vi "Supervisor Chat.vi"(9 "Stop Chat":bool, 10 "Send":bool, 11 "Enter Text":string) -> (3 "Chat Window":string)   [LabVIEW 2017]
uses:
  <vilib>/OPCUA/controls/Write Status.ctl
  <vilib>/OPCUA/controls/NodeId.ctl
  <vilib>/OPCUA/client/Multiple Write String.vi
  <vilib>/OPCUA/NI OPC UA Client.lvlib
panel:
  out "Log Loop":i32
  out "Send Loop":i32
  in  "Node Status":T1 items=["Good"=0, "Uncertain_InitialValue"=1083310080, "Uncertain_LastUsableValue"=1083179008, "Uncertain_SensorNotAccurate"=1083375616, "Uncertain_EngineeringUnitsExceeded"=1083441152, "Bad_NoCommunication"=2150694912, "Bad_NotReadable"=2151284736, "Bad_NotWritable"=2151350272, "Bad_OutOfRange"=2151415808, "Bad_WaitingForInitialData"=2150760448]
  in  "Time Stamp":timestamp
  in  "Node Status":T1 items=["Good"=0, "Uncertain_InitialValue"=1083310080, "Uncertain_LastUsableValue"=1083179008, "Uncertain_SensorNotAccurate"=1083375616, "Uncertain_EngineeringUnitsExceeded"=1083441152, "Bad_NoCommunication"=2150694912, "Bad_NotReadable"=2151284736, "Bad_NotWritable"=2151350272, "Bad_OutOfRange"=2151415808, "Bad_WaitingForInitialData"=2150760448]
  in  "Time Stamp":timestamp
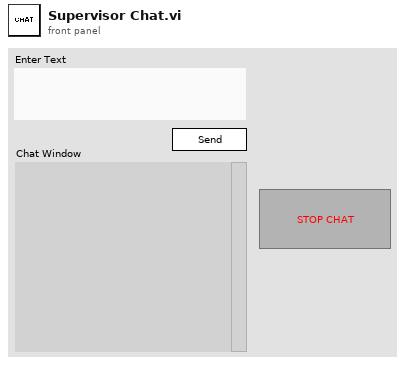
[diagram p1: front panel]
types:
  T1 = typedef "Write Status.ctl" = u32
  T2 = enum16{"open", "replace", "create", "open or create", "replace or create", "replace or create with confirmation"}
  T3 = typedef "OPC UA Client Refnum.ctl" = refnum<k21>
  T4 = typedef "NodeId.ctl" = string
  T5 = cluster{"node ID":T4, "value":string, "timestamp (current time)":timestamp, "node status":T1}
  T6 = cluster{"node ID":T4, "value":string, "timestamp (current time)":timestamp, "node status":T1}[]
  T7 = typedef "Subscription ID.ctl" = u32
  T8 = typedef "Subscription Data Change.ctl" = cluster{"node ID":T4, " value":variant, "timestamp":timestamp, "data type":T9, "status code":T10}
  T9 = typedef "Data Type.ctl" = u16
  T10 = typedef "OPC UA StatusCode.ctl" = u32
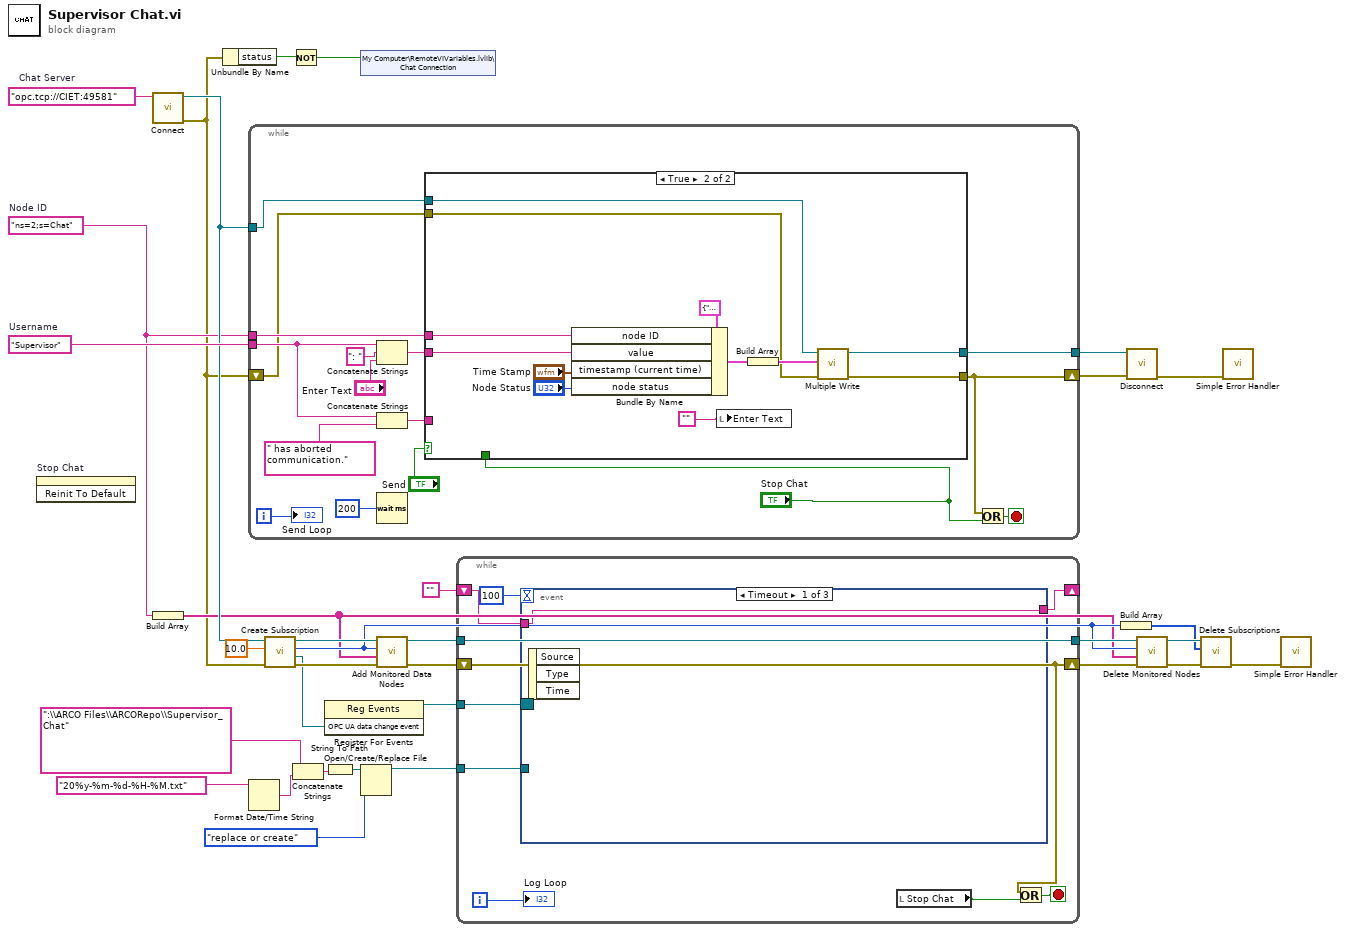
[diagram p0: block diagram]
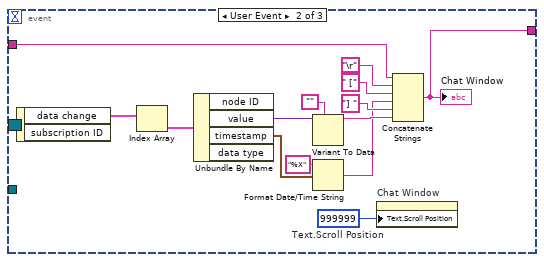
[diagram p2: hidden frame]
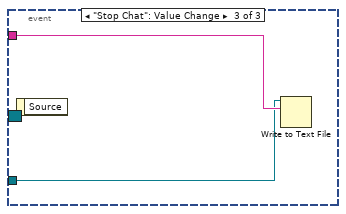
[diagram p3: hidden frame]
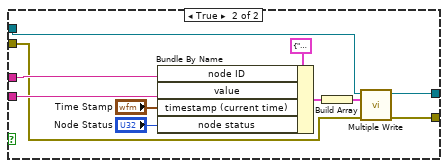
[diagram p5: hidden frame]
diagram:
  w15 = "ns=2;s=Chat"  # Node ID
  w31 = "Supervisor"  # Username
  w32 = "opc.tcp://CIET:49581"  # Chat Server
  n1 = invoke on="Stop Chat" class="Bool (strict)" method="Reinit To Default"() -> ()  [unwired: 3 in, 3 out]
  n2 = call <vilib>:"Connect.vi"("server endpoint URL"=w32) -> ("error out"=w3:errorcluster, "OPC UA client refnum out"=w30:T3)  [unwired: 8 in, 1 out]
  n3 = Build Array(w15) -> (w14:string[])
  n4 = Unbundle By Name(w3) -> ("status"=w5:bool)
  n5 = while {
    tunnel: w15 -> [w41]
    tunnel: w31 -> [w46]
    tunnel: w30 -> [w39]
    tunnel: [w40] -> w12
    shift-right: [w34] -> w2
    shift-left: w3 -> [w38]
    i -> [w44]
    stop <- w36 stop-if-true
    n6 = Concatenate Strings(w46, ": ", "Enter Text") -> (w42:string)
    n7 = Concatenate Strings(w46, " has aborted communication.") -> (w37:string)
    n8 = Wait (ms)(milliseconds to wait=u32 200) -> ()  [unwired: 1 out]
    n9 = case shown="True" "Send" {
      tunnel: w42 -> [_ w76]
      tunnel: w41 -> [w54 w75]
      tunnel: [w50 w73] -> w40
      tunnel: [w51 w72] -> w34
      tunnel: w39 -> [w52 w71]
      tunnel: w38 -> [w53 w70]
      tunnel: "Stop Chat" -> [w56 _]
      tunnel: w37 -> [w55 _]
      frame False {
        n10 = case shown="False" w56 {
          tunnel: w55 -> [_ w64]
          tunnel: w54 -> [_ w63]
          tunnel: w53 -> [w57 w62]
          tunnel: w52 -> [w58 w61]
          tunnel: [w58 w60] -> w50
          tunnel: [w57 w59] -> w51
          frame False {
          }
          frame True {
            n11 = Bundle By Name(cluster=T5 {"node ID"="", "value"="", "timestamp (current time)"=timestamp(0 s since 1904-01-01), "node status"=0} ("request"), "node ID"=w63, "value"=w64, "timestamp (current time)"="Time Stamp", "node status"="Node Status") -> (w67:T5)
            n12 = Build Array(w67) -> (w66:T6)
            n13 = call-poly <vilib>:"Multiple Write.vi"("error in (no error)"=w62, "requests"=w66, "OPC UA client refnum in"=w61) -> ("error out"=w59:errorcluster, "OPC UA client refnum out"=w60:T3)  [unwired: 5 in, 2 out]
          }
        }
      }
      frame True {
        n14 = Bundle By Name(cluster=T5 {"node ID"="", "value"="", "timestamp (current time)"=timestamp(0 s since 1904-01-01), "node status"=0} ("request"), "node ID"=w75, "value"=w76, "timestamp (current time)"="Time Stamp", "node status"="Node Status") -> (w79:T5)
        n15 = local write "Enter Text"("") -> ()
        n16 = Build Array(w79) -> (w78:T6)
        n17 = call-poly <vilib>:"Multiple Write.vi"("error in (no error)"=w70, "requests"=w78, "OPC UA client refnum in"=w71) -> ("error out"=w72:errorcluster, "OPC UA client refnum out"=w73:T3)  [unwired: 5 in, 2 out]
      }
    }
    n18 = Or(x=w34, y="Stop Chat") -> (x .or. y?=w36:bool)
    "Send Loop" <- w44
  }
  n19 = Format Date/Time String(time format string (%c)="20%y-%m-%d-%H-%M.txt") -> (date/time string=w9:string)  [unwired: 2 in]
  n20 = call <vilib>:"Create Subscription.vi"("error in (no error)"=w3, "publishing interval (1000 ms)"=10.0, "OPC UA client refnum in"=w30) -> ("error out"=w28:errorcluster, "OPC UA data change event"=w27:refnum<user-event>, "subscription ID out"=w19:T7, "OPC UA client refnum out"=w29:T3)  [unwired: 4 in, 1 out]
  n21 = Not(x=w5) -> (.not. x?=w4:bool)
  n22 = Concatenate Strings(":\\ARCO Files\\ARCORepo\\Supervisor_Chat", w9) -> (w7:string)
  n23 = register-events(w27) -> (reference out=w26:refnum<event-registration>)  [unwired: 2 in, 1 out]
  n24 = String To Path(string=w7) -> (path=w6:path)
  n25 = shared-variable "My Computer\\RemoteVIVariables.lvlib\\Chat Connection"(w4) -> ()  [unwired: 1 in, 1 out]
  n26 = Open/Create/Replace File(file path (use dialog)=w6, operation (0:open)=T2."replace or create") -> (refnum out=w16:refnum<file>)  [unwired: 4 in, 2 out]
  n27 = call <vilib>:"Add Monitored Data Nodes.vi"("error in (no error)"=w28, "node IDs"=w14, "subscription ID in"=w19, "OPC UA client refnum in"=w29) -> ("error out"=w22:errorcluster, "OPC UA client refnum out"=w24:T3)  [unwired: 4 in, 2 out]
  n28 = while {
    tunnel: w26 -> [w91]
    shift-right: [w89] -> _
    shift-left: "" -> [w90]
    tunnel: w24 -> [w88]
    tunnel: [w88] -> w23
    tunnel: w16 -> [w87]
    shift-right: [w83] -> w1
    shift-left: w22 -> [w83]
    i -> [w86]
    stop <- w84 stop-if-true
    n29 = event shown="[0] Timeout" {
      selector: w91 -> [_ _ _]
      dyn-events: _ -> [_ _ _]
      timeout: 100 -> [_ _ _]
      tunnel: w90 -> [w92 w95 w108]
      tunnel: [w92 w94 _] -> w89
      tunnel: w87 -> [_ _ w107]
      event Timeout {
        n30 = event-data() -> ()  [unwired: 1 in, 3 out]
      }
      event User Event {
        w93 = u32 999999  # Text.Scroll Position
        n31 = event-data() -> ("data change"=w106:T8[])  [unwired: 1 in, 1 out]
        n32 = Index Array(array=w106) -> (element=w105:T8)  [unwired: 1 in]
        n33 = Unbundle By Name(w105) -> ("value"=w104:variant, "timestamp"=w102:timestamp)  [unwired: 2 out]
        n34 = Variant To Data(type="", Variant=w104) -> (data=w100:string)  [unwired: 1 in, 1 out]
        n35 = Format Date/Time String(time format string (%c)="%X", seconds (now)=w102) -> (date/time string=w98:string)  [unwired: 1 in]
        n36 = property on="Chat Window" class="Str"("Text.Scroll Position"=w93) -> ()  [unwired: 2 in, 2 out]
        n37 = Concatenate Strings(w95, "\r", " [", w98, "] ", w100) -> (w94:string)
        "Chat Window" <- w94
      }
      event "Stop Chat": Value Change {
        n38 = event-data() -> ()  [unwired: 1 in, 1 out]
        n39 = Write to Text File(file (use dialog)=w107, text=w108) -> ()  [unwired: 2 in, 3 out]
      }
    }
    n40 = local read "Stop Chat"() -> (w82:bool)
    n41 = Or(x=w83, y=w82) -> (x .or. y?=w84:bool)
    "Log Loop" <- w86
  }
  n42 = Build Array(w19) -> (w18:T7[])
  n43 = call <vilib>:"Disconnect.vi"("error in (no error)"=w2, "OPC UA client refnum in"=w12) -> ("error out"=w33:errorcluster)  [unwired: 9 in]
  n44 = call <vilib>:"Delete Monitored Nodes.vi"("error in (no error)"=w1, "node IDs"=w14, "subscription ID in"=w19, "OPC UA client refnum in"=w23) -> ("error out"=w20:errorcluster, "OPC UA client refnum out"=w21:T3)  [unwired: 3 in, 3 out]
  n45 = call <vilib>:"Delete Subscriptions.vi"("error in (no error)"=w20, "subscription IDs"=w18, "OPC UA client refnum in"=w21) -> ("error out"=w17:errorcluster)  [unwired: 6 in, 2 out]
  n46 = call <vilib>:"Simple Error Handler.vi"("error in (no error)"=w33) -> ()  [unwired: 4 in, 5 out]
  n47 = call <vilib>:"Simple Error Handler.vi"("error in (no error)"=w17) -> ()  [unwired: 4 in, 5 out]
